vi "Set Entry Mode.vi"(6 "chip select  (1st chip)":enum16{"1st chip", "2nd chip"}(ring), 8 "error in (no error)":errorcluster, 10 "entry mode":T1(ring), 11 "Character LCD in":refnum<class "Character LCD.lvclass">) -> (0 "error out":errorcluster, 3 "Character LCD out":refnum<class "Character LCD.lvclass">)   [LabVIEW 2017, in "Character LCD.lvclass"]
uses:
  Character LCD.lvclass
  Common/HD44780 Common.lvlib
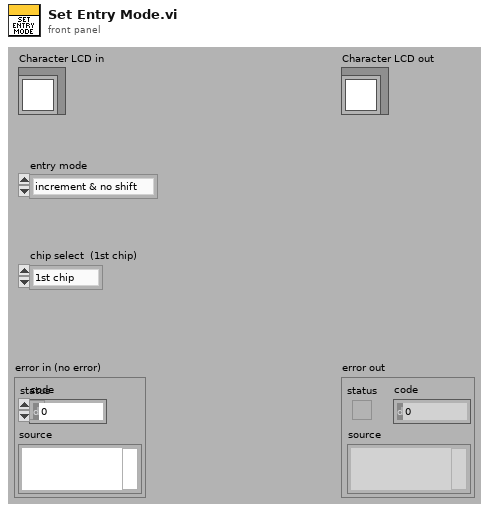
[diagram p1: front panel]
types:
  T1 = enum8{"increment & no shift", "increment & shift", "decrement & no shift", "decrement & shift"}
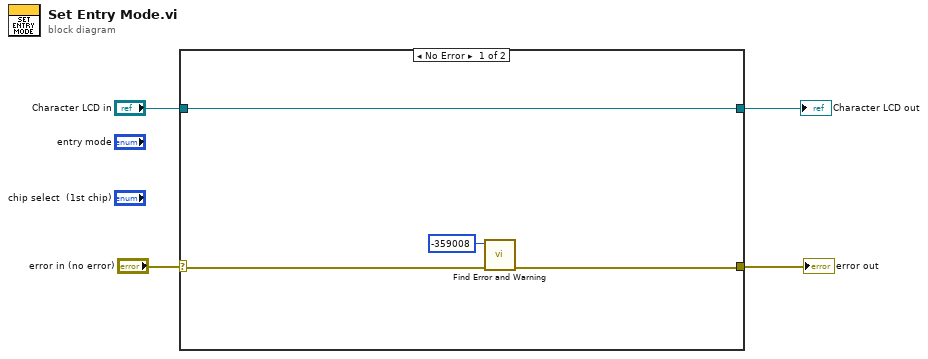
[diagram p0: block diagram]
diagram:
  n1 = case shown="No Error" "error in (no error)" {
    selector: "error in (no error)" -> [w6 w10]
    tunnel: [w5 w10] -> w3
    tunnel: [w8 w9] -> w1
    tunnel: "Character LCD in" -> [w8 w9]
    frame No Error {
      n2 = call "Find Error and Warning.vi"("error in (no error)"=w6, "error code"=-359008) -> ("error out"=w5:errorcluster)  [unwired: 9 in]
    }
    frame Error {
    }
  }
  "error out" <- w3
  "Character LCD out" <- w1
